vi "TimerOffDelay.vi"(10 "Time Delay":u32, 11 "Input":bool) -> (3 "Output":bool)   [LabVIEW 2016]
doc: "Output becomes true Time Limit ms after Input becomes true and stays true"
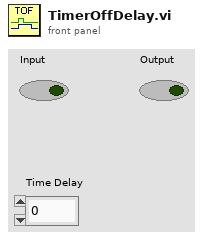
[diagram p1: front panel]
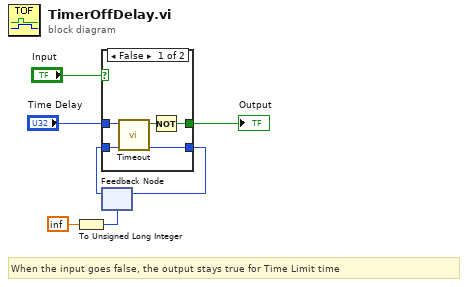
[diagram p0: block diagram]
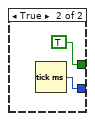
[diagram p2: hidden frame]
diagram:
  # "When the input goes false, the output stays true for Time Limit time"
  n1 = To Unsigned Long Integer(number=inf) -> (unsigned 32bit integer=w4:u32)
  n2 = feedback #1(w4) -> (w6:u32)
  n3 = case shown="False" "Input" {
    tunnel: [w8 TRUE ("Output")] -> w1
    tunnel: [w11 w13] -> w7
    tunnel: w6 -> [w12 _]
    tunnel: "Time Delay" -> [w10 _]
    frame False {
      n4 = call "Timeout.vi"("Start Time In"=w12, "Time Limit (ms)"=w10) -> ("Start Time Out"=w11:u32, "Timeout"=w9:bool)  [unwired: 8 in]
      n5 = Not(x=w9) -> (.not. x?=w8:bool)
    }
    frame True {
      n6 = Tick Count (ms)() -> (millisecond timer value=w13:u32)
    }
  }
  "Output" <- w1
  n7 = feedback-in #1(w7) -> ()
